vi "chart axis set label position.vi"(8 "error in (no error)":errorcluster, 10 "position":u8, 11 "axis":u32) -> (0 "error out":errorcluster)   [LabVIEW 8.6]
doc: "void chart_axis_set_label_position(lxw_chart_axis axis, uint8_t position);"
uses:
  pending_lvxlsxwriter/xlsxwriter.dll
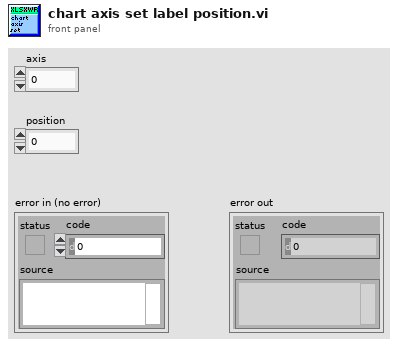
[diagram p1: front panel]
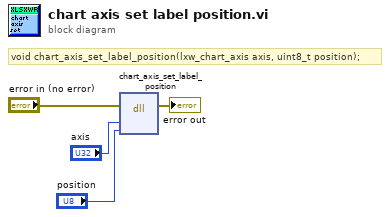
[diagram p0: block diagram]
diagram:
  # "void chart_axis_set_label_position(lxw_chart_axis axis, uint8_t position);"
  n1 = dll-call lib="C:/Users/WDAGUtilityAccount/Desktop/pending_lvxlsxwriter/xlsxwriter.*" fn="chart_axis_set_label_position"(error in="error in (no error)", "axis"="axis", "position"="position") -> (error out=→"error out":errorcluster)  [unwired: 5 in, 1 out]
